vi "Bookmark Diagram Disable Structure.vi"(8 "Error In":errorcluster, 11 "DisableStructure In":refnum<vi>) -> (0 "Error Out":errorcluster, 3 "DisableStructure Out":refnum<vi>)   [LabVIEW 2017, in "Eulogy.lvlib"]
uses:
  Eulogy.lvlib
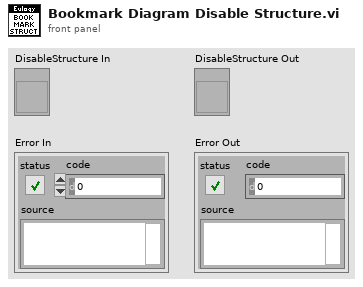
[diagram p1: front panel]
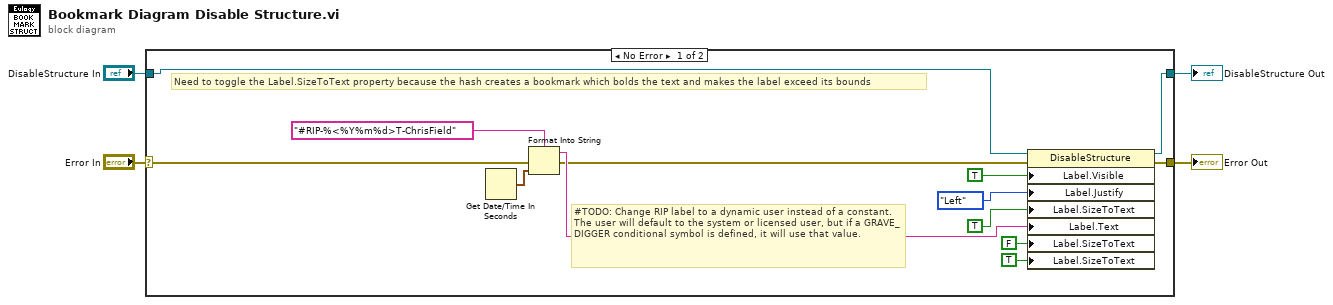
[diagram p0: block diagram]
diagram:
  n1 = case shown="No Error" "Error In" {
    selector: "Error In" -> [w5 w18]
    tunnel: [w13 w19] -> w4
    tunnel: [w12 w18] -> w3
    tunnel: "DisableStructure In" -> [w11 w19]
    frame No Error {
      # "#TODO: Change RIP label to a dynamic user instead of a constant. The user will default to the system or licensed user, but if a GRAVE_DIGGER conditional symbol is defined, it will use that value."
      # "Need to toggle the Label.SizeToText property because the hash creates a bookmark which bolds the text and makes the label exceed its bounds"
      n2 = Get Date/Time In Seconds() -> (seconds since 1Jan1904=w15:timestamp)
      n3 = Format Into String(format string="#RIP-%<%Y%m%d>T-ChrisField", error in=w5, w15) -> (resulting string=w17:string, error out=w16:errorcluster)  [unwired: 1 in]
      n4 = property class="DisableStructure"(reference=w11, error in=w16, "Label.Visible"=TRUE ("Label.Size to Text?"), "Label.Justify"=enum16{"Left", "Center", "Right"}."Left" ("Label.Justification"), "Label.SizeToText"=TRUE ("Label.Size to Text?"), "Label.Text"=w17, "Label.SizeToText"=FALSE ("Label.Size to Text?"), "Label.SizeToText"=TRUE ("Label.Size to Text?")) -> (reference out=w13:refnum<vi>, error out=w12:errorcluster)
    }
    frame Error {
    }
  }
  "DisableStructure Out" <- w4
  "Error Out" <- w3
